vi "Process_data.vi"(4 "Measurement top level?":bool) -> (6 "Vel stat display":string[][](table), 7 "First Plot data Cluster":cluster{"X array":dbl[], "Y array":dbl[]}[](array[cluster]), 8 "Second Plot Data Cluster":cluster{"X array":dbl[], "Y array":dbl[]}[](array[cluster]), 9 "Max Measurement time up":bool)   [LabVIEW 2014]
uses:
  Controls/Inst_type.ctl
  Controls/Instrument_Array.ctl
  Controls/Post_Process.ctl
  Controls/User_Specific_mode.ctl
  Globals/Meas_global.vi
  Globals/LDA_meas_global_1.vi
  Acquisition/PWA/PWAtasksGLOBAL.vi
  Globals/Dynamic_call_global.ph.vi
  Globals/Trav_pos_global.vi
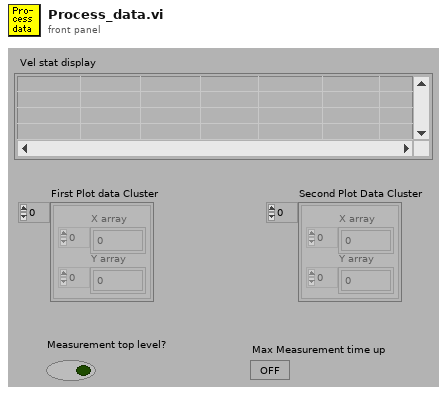
[diagram p1: front panel]
types:
  T1 = typedef "LDA_Setup.ctl" = cluster{"dimensions":enum16{"1D", "2D"}, "Analogue Freq Multiplier":dbl}
  T2 = typedef "PWA_Data.ctl" = enum16{"No PWA Data", "One Ch PWA"}
  T3 = typedef "Inst_type.ctl" = enum16{"Propeller anemometer", "Raw voltage", "Pressure Transducer", "Pitot-static tube", "Preston tube", "Hot wire", "Cross wire 1", "Cross wire 2", "Generic Linear", "Generic Polynomial", "Generic BackPoly", "Fast FID", "Thermocouple", "Cold wire", "Pulsed Wire", "LDA Vel", "LDA Tran time", "LDA Arr time", "Microphone"}
  T4 = typedef "Instrument_Array.ctl" = enum16{"PWA", "LDA", "Analogue"}
  T5 = typedef "Post_Process.ctl" = enum16{"Take New Data", "Post Process Raw Data File"}
  T6 = typedef "User_Specific_mode.ctl" = enum16{"Check VI only", "Run VI"}
  T7 = typedef "Trigger_Mode.ctl" = enum16{"Free Running", "Start on Trigger", "Trigger Every Block", "Trigger Every Sample"}
  T8 = typedef "Analysis_info_cluster.ctl" = cluster{"Colour":u32, "Inst type":T3, "Inst name":string, "Symbol":string, "Code name":string, "Extra Info":string, "Inst Array":T4, "Extra Titles":string[], "Extra Values":string[], "U":dbl, "u^2":dbl, "u^3":dbl, "u^4":dbl, "Skew_u":dbl, "Kurt_u":dbl, "Sd Error in Mean":dbl, "% u'/U":dbl, "X":dbl, "Y":dbl, "Z":dbl, "Timescale integral to 25%":dbl, "Sd Error in Variance":dbl, "Calib File":path, "Calib Constants":dbl[], "Output Position":bool, "Full Stats":bool, "Av Sampling Rate":dbl, "Av No of Samples":dbl, "Total Meas Time (s)":dbl, "ADAM Ch Name":string}
  T9 = typedef "Time_Trace_Cluster.ctl" = cluster{"Weighting":dbl[], "Time (s)":dbl[], "Voltage":dbl[], "Eng Values":dbl[]}
  T10 = typedef "Shift_Cluster.ctl" = cluster{"Stats":dbl[], "Spectra_Auto":dbl[], "Histogram":dbl[], "Hist Max":dbl, "Hist Min":dbl, "No of Samples":i32, "No in plume":i32, "Weigth sum":dbl}
  T11 = typedef "Correlation_cluster1.ctl" = cluster{"U inst":string, "uw":dbl, "u^2w":dbl, "uw^2":dbl, "uw/u'w'":dbl, "W inst":string, "uw^3":dbl, "u^3w":dbl, "u^2w^2":dbl, "Index U":i32, "Index W":i32}
  T12 = typedef "Traverse_cluster.ctl" = cluster{"Start X":sgl, "Start Y":sgl, "Start Z":sgl, "End X":sgl, "End Y":sgl, "End Z":sgl, "No. of pts.":i32, "Spacing":T13, "Filename":path, "Tunnel Speed":dbl, "Averaging time (min)":dbl, "Extra Commands":string, "Carrier_1 Q (l/min)":dbl, "Carrier_2 Q (l/min)":dbl, "Trace Gas Concentration (%)":dbl, "Specific Arguments":string, "Comments":string, "Row No":i32, "Row Type Selector":T14, "Completion time":string, "Row Duration (mins)":dbl, "No. of Valid pts.":i32, "Meas Setup File":string}
  T13 = typedef "Spacing.ctl" = enum16{"Linear", "Log", "Gauss", "Specified", "N/A"}
  T14 = typedef "Multi_run_mode.ctl" = enum16{"Move Traverse Only", "Set Tunnel Speed Only", "Set Source Only", "Set Measurement Conditions", "Single Measurement", "Vertical Profile", "Lateral Profile", "Longitudinal Profile", "Explore Volume", "Multi-Axis Profile", "Auto Calibrate", "Meas Fast FID Bkgnd", "Check Beam Power", "Scanning Valve Measurement", "Run VI Named:", "Set ADAM Ch", "Wait (minutes)", "Send Message", "Synchronize With:", "Fall Back to this Row", "Turn Off Row Repeating", "Blank Row", "Traverse 3D Volume"}
  T15 = typedef "Graph_Type.ctl" = enum16{"Show no graph", "Voltage trace", "Velocity trace", "Vel histogram", "Spectrum", "f.E(f) v Log f", "Auto-Corr"}
  T16 = cluster{"Plot 1":u16, "Plot 2":u16, "Save graph":u16, "Plot Type":T15}
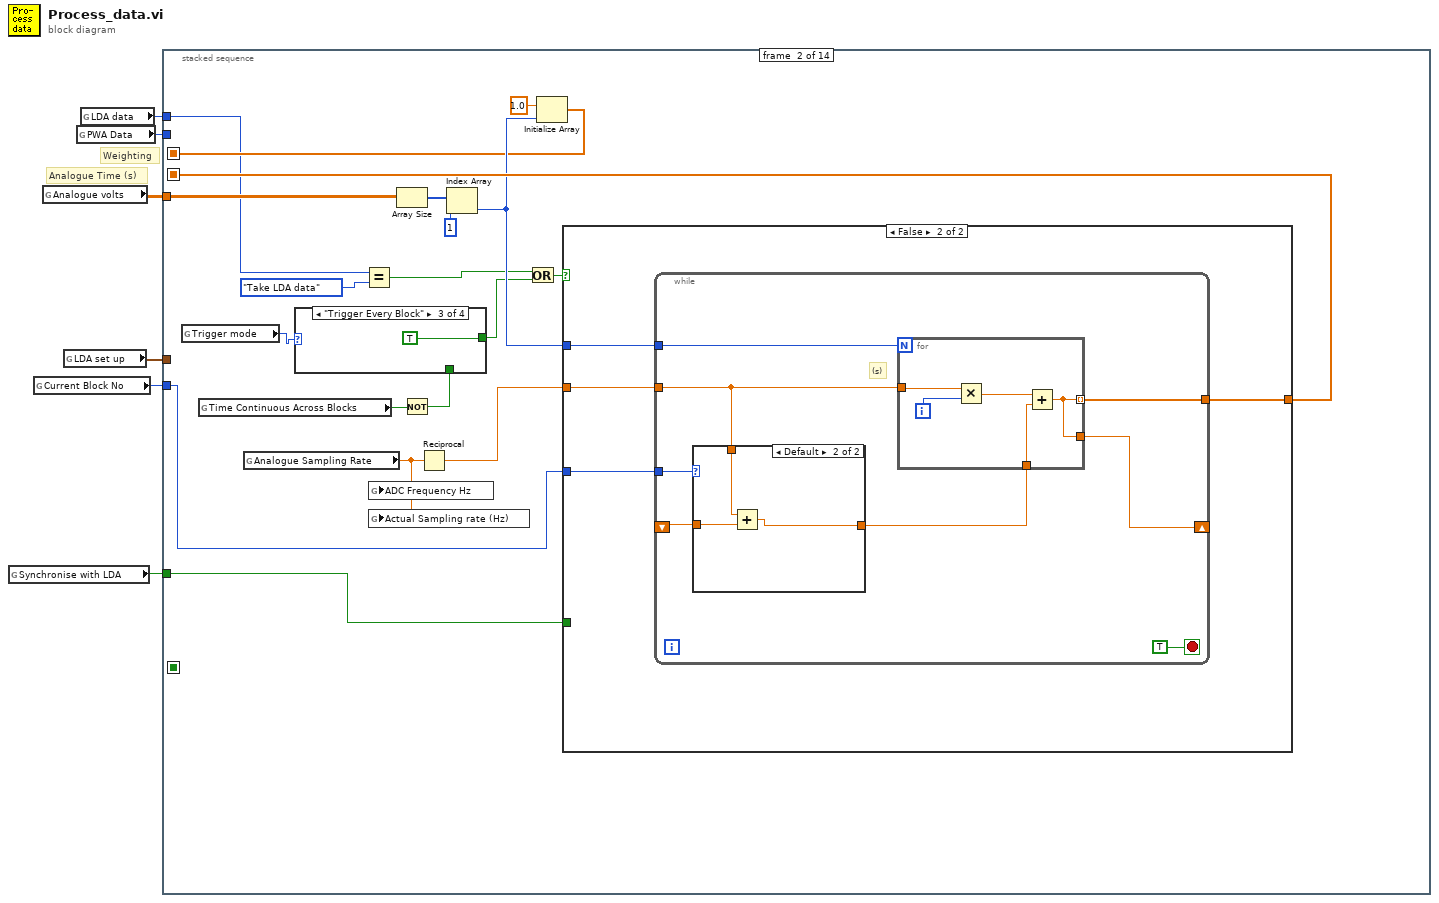
[diagram p0: block diagram]
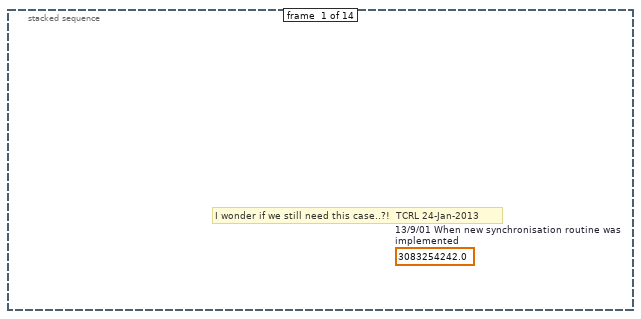
[diagram p2: hidden frame]
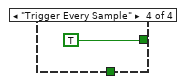
[diagram p5: hidden frame]
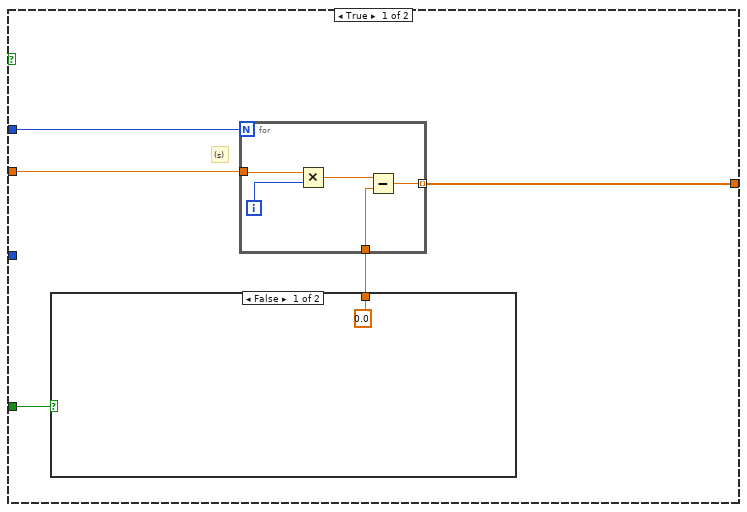
[diagram p6: hidden frame]
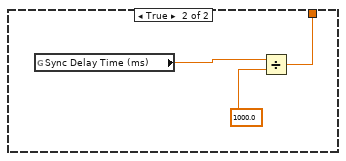
[diagram p7: hidden frame]
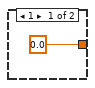
[diagram p8: hidden frame]
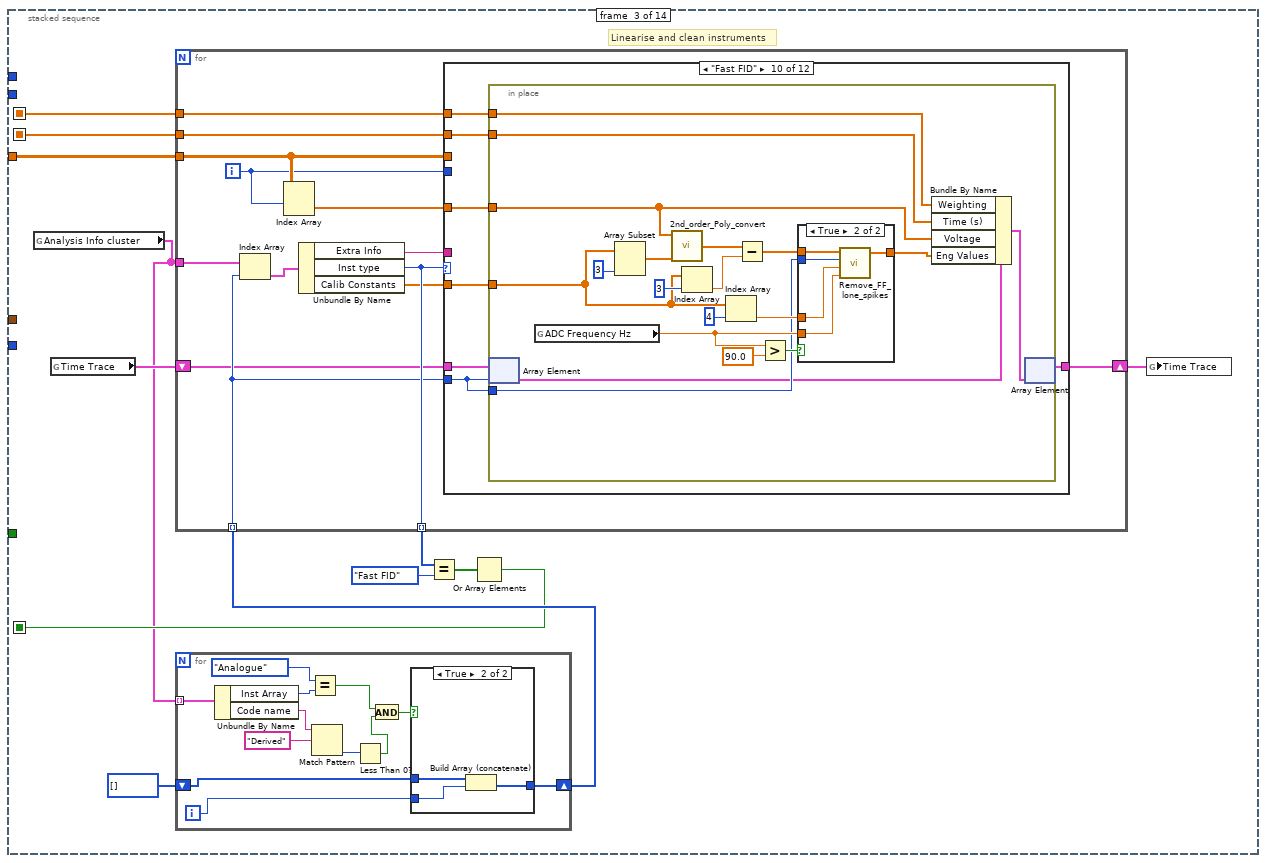
[diagram p9: hidden frame]
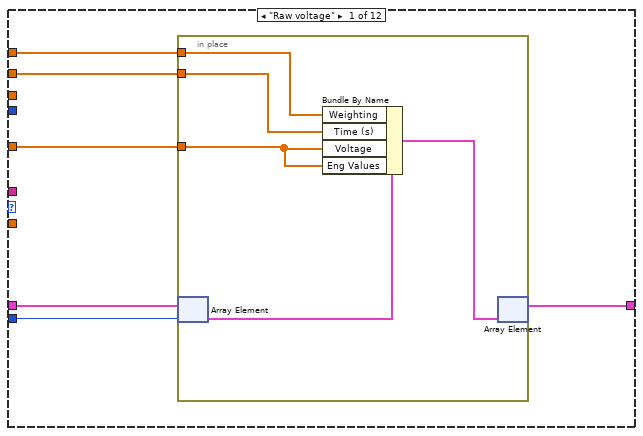
[diagram p11: hidden frame]
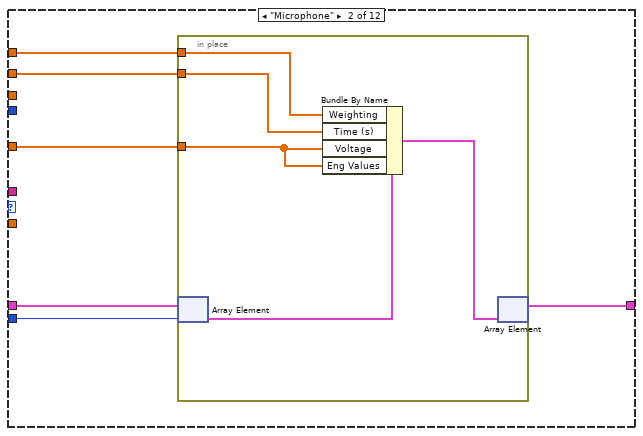
[diagram p12: hidden frame]
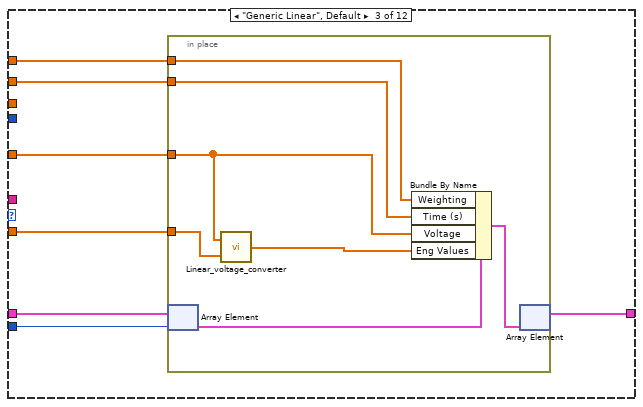
[diagram p13: hidden frame]
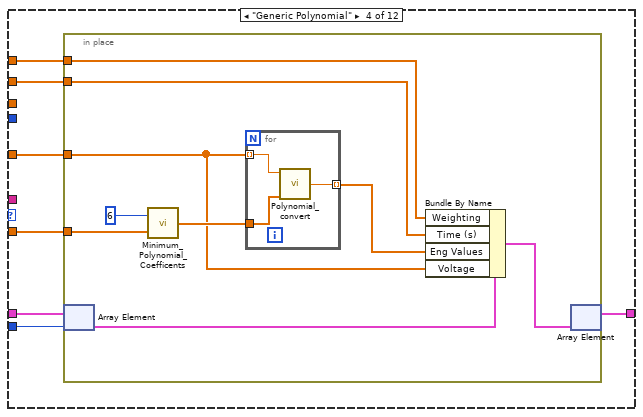
[diagram p14: hidden frame]
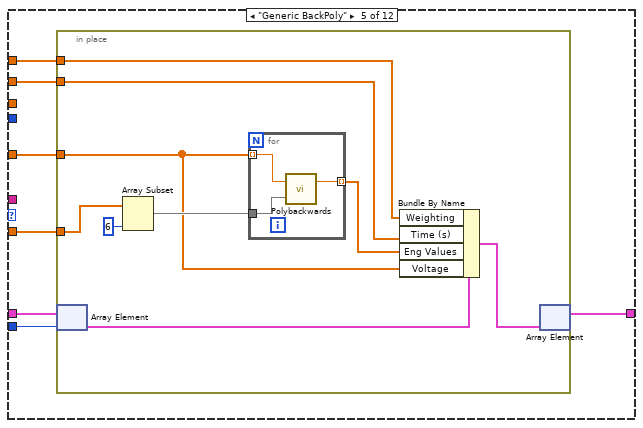
[diagram p15: hidden frame]
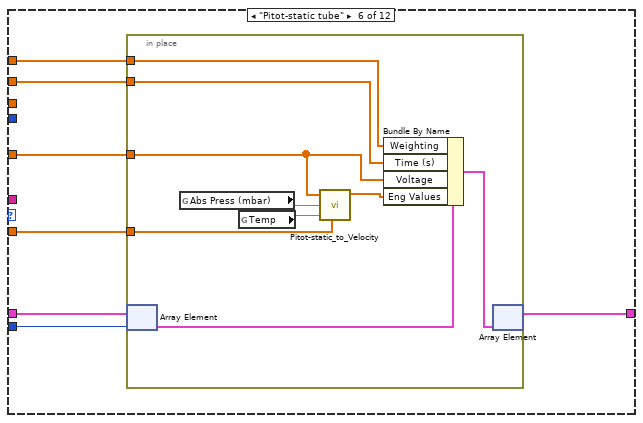
[diagram p16: hidden frame]
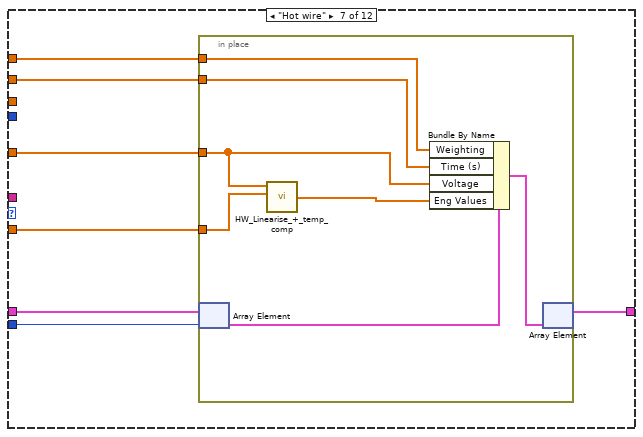
[diagram p17: hidden frame]
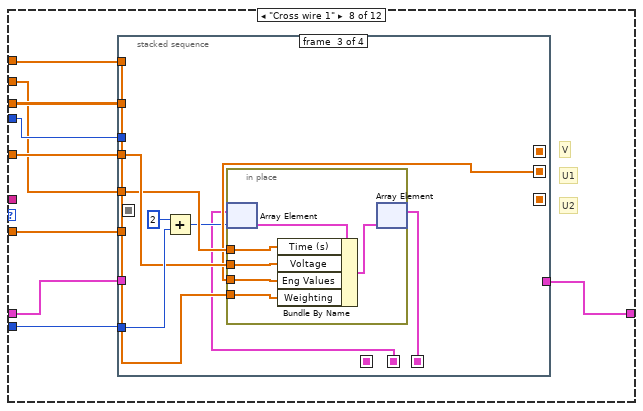
[diagram p18: hidden frame]
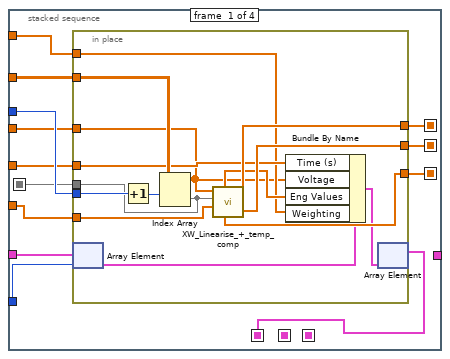
[diagram p19: hidden frame]
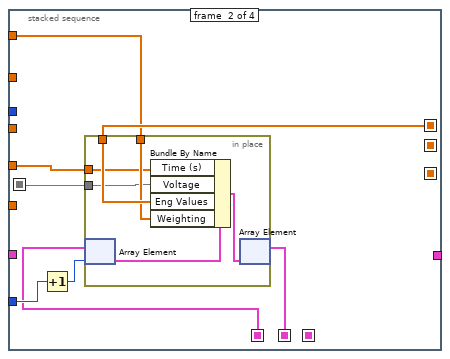
[diagram p20: hidden frame]
diagram:
  # "Weighting"
  # "Analogue Time (s)"
  n1 = global read "Meas_global.vi" "Synchronise with LDA"() -> (w4:bool)
  n2 = global read "Meas_global.vi" "Current Block No"() -> (w5:i32)
  n3 = global read "Meas_global.vi" "Analogue volts"() -> (w2:dbl[][])
  n4 = global read "Meas_global.vi" "LDA set up"() -> (w1:T1)
  n5 = global read "Meas_global.vi" "PWA Data"() -> (w3:T2)
  n6 = global read "Meas_global.vi" "LDA data"() -> (w6:enum16{"No LDA data", "Take LDA data"})
  n7 = stacked-sequence {
    seq-local: [_ w22 _ _ _ _ _ _ _ _ _ _ _ _] -> [_ _ w70 _ _ _ _ _ _ _ _ _ _ _]
    seq-local: [_ w19 _ _ _ _ _ _ _ _ _ _ _ _] -> [_ _ w69 _ _ _ _ _ _ _ _ _ _ _]
    seq-local: [_ _ w66 _ _ _ _ _ _ _ _ _ _ _] -> [_ _ _ _ w431 _ _ _ _ _ _ _ _ _]
    tunnel: w5 -> [_ w15 _ _ _ w435 _ _ _ _ _ _ _ _]
    tunnel: w6 -> [_ w12 _ w385 _ _ _ _ _ _ _ _ _ _]
    tunnel: w2 -> [_ w25 w76 _ _ _ _ _ _ _ _ w644 _ _]
    tunnel: w4 -> [_ w16 _ w384 _ _ _ _ _ _ _ _ _ _]
    tunnel: w3 -> [_ _ _ _ _ w438 _ _ _ _ _ _ _ _]
    tunnel: w1 -> [_ _ _ w382 _ _ _ _ _ _ _ _ _ _]
    frame #0 {
      (unwired) 3083254242.0  # 13/9/01 When new synchronisation routine was implemented
      # "I wonder if we still need this case..?!  TCRL 24-Jan-2013"
    }
    frame #1 {
      n8 = global read "Meas_global.vi" "Trigger mode"() -> (w14:T7)
      n9 = global read "Meas_global.vi" "Time Continuous Across Blocks"() -> (w8:bool)
      n10 = global read "Meas_global.vi" "Analogue Sampling Rate"() -> (w18:dbl)
      n11 = Equal?(x=w12, y=enum16{"No LDA data", "Take LDA data"}."Take LDA data" ("LDA data")) -> (x = y?=w10:bool)
      n12 = global write "LDA_meas_global_1.vi" "ADC Frequency Hz"(w18) -> ()
      n13 = global write "Meas_global.vi" "Actual Sampling rate (Hz)"(w18) -> ()
      n14 = Array Size(array=w25) -> (size(s)=w24:i32[])
      n15 = Not(x=w8) -> (.not. x?=w7:bool)
      n16 = case shown="\"Trigger Every Block\"" w14 {
        tunnel: [w26 w27 TRUE TRUE] -> w9
        tunnel: w7 -> [w26 w27 _ _]
        frame "Free Running" {
        }
        frame "Start on Trigger" {
        }
        frame "Trigger Every Block" {
        }
        frame "Trigger Every Sample" {
        }
      }
      n17 = Reciprocal(x=w18) -> (1/x=w17:dbl)
      n18 = Index Array(array=w24, index=1) -> (element=w21:i32)
      n19 = Or(x=w10, y=w9) -> (x .or. y?=w11:bool)
      n20 = Initialize Array(1.0 ("element"), w21) -> (w19:dbl[])
      n21 = case shown="False" w11 {
        tunnel: [w34 w47] -> w22
        tunnel: w21 -> [w33 w46]
        tunnel: w17 -> [w31 w45]
        tunnel: w16 -> [w30 _]
        tunnel: w15 -> [_ w44]
        frame True {
          # "(s)"
          n22 = case shown="False" w30 {
            tunnel: [0.0 w37] -> w32
            frame False {
            }
            frame True {
              n23 = global read "LDA_meas_global_1.vi" "Sync Delay Time (ms)"() -> (w38:dbl)
              n24 = Divide(x=w38, y=1000.0) -> (x/y=w37:dbl)
            }
          }
          n25 = for {
            N: w33 -> [_]
            tunnel: w31 -> [w42]
            tunnel: [w41] -> w34 mode=indexing
            tunnel: w32 -> [w39]
            i -> [w43]
            n26 = Multiply(x=w42, y=w43) -> (x*y=w40:dbl)
            n27 = Subtract(x=w40, y=w39) -> (x-y=w41:dbl)
          }
        }
        frame False {
          n28 = while {
            tunnel: [w55] -> w47
            tunnel: w46 -> [w54]
            tunnel: w45 -> [w48]
            tunnel: w44 -> [w52]
            shift-right: [w50] -> _
            shift-left: _ -> [w49]
            stop <- TRUE stop-if-true
            # "(s)"
            n29 = case shown="Default" w52 {
              tunnel: [0.0 w57] -> w51
              tunnel: w49 -> [_ w59]
              tunnel: w48 -> [_ w58]
              frame 1 {
              }
              frame Default {
                n30 = Add(x=w58, y=w59) -> (x+y=w57:dbl)
              }
            }
            n31 = for {
              N: w54 -> [_]
              tunnel: w48 -> [w63]
              tunnel: [w60] -> w55 mode=indexing
              tunnel: w51 -> [w61]
              tunnel: [w60] -> w50
              i -> [w64]
              n32 = Multiply(x=w63, y=w64) -> (x*y=w62:dbl)
              n33 = Add(x=w62, y=w61) -> (x+y=w60:dbl)
            }
          }
        }
      }
    }
    frame #2 {
      # "Linearise and clean instruments"
      n34 = global read "Meas_global.vi" "Analysis Info cluster"() -> (w65:T8[])
      n35 = global read "Meas_global.vi" "Time Trace"() -> (w68:T9[])
      n36 = for {
        tunnel: w65 -> [w80] mode=indexing
        shift-right: [w77] -> w71
        shift-left: i32[] [] -> [w78]
        i -> [w79]
        n37 = Unbundle By Name(w80) -> ("Inst Array"=w88:T4, "Code name"=w86:string)
        n38 = Equal?(x=Instrument_Array."Analogue" ("Inst Array"), y=w88) -> (x = y?=w82:bool)
        n39 = Match Pattern(string=w86, regular expression="Derived") -> (offset past match=w84:i32)  [unwired: 4 out]
        n40 = Less Than 0?(x=w84) -> (x < 0?=w83:bool)
        n41 = And(x=w82, y=w83) -> (x .and. y?=w81:bool)
        n42 = case shown="True" w81 {
          tunnel: w79 -> [_ w92]
          tunnel: w78 -> [w89 w91]
          tunnel: [w89 w90] -> w77
          frame False {
          }
          frame True {
            n43 = Build Array (concatenate)(w91, w92) -> (w90:i32[])
          }
        }
      }
      n44 = for {
        tunnel: w76 -> [w104]
        tunnel: [w105] -> w74 mode=indexing
        tunnel: w71 -> [w100] mode=indexing
        shift-right: [w95] -> w67
        shift-left: w68 -> [w99]
        tunnel: w70 -> [w96]
        tunnel: w69 -> [w103]
        tunnel: w65 -> [w102]
        i -> [w94]
        n45 = Index Array(array=w102, index=w100) -> (element=w101:T8)
        n46 = Index Array(array=w104, index (row)=w94) -> (element=w98:dbl[])  [unwired: 1 in]
        n47 = Unbundle By Name(w101) -> ("Extra Info"=w93:string, "Inst type"=w105:T3, "Calib Constants"=w97:dbl[])
        n48 = case shown="\"Fast FID\"" w105 {
          tunnel: w97 -> [_ _ w134 w147 w167 w186 w202 w217 _ w297 w328 w365]
          tunnel: w94 -> [_ _ _ _ _ _ _ w218 _ _ _ _]
          tunnel: w104 -> [_ _ _ _ _ _ _ w215 _ _ _ _]
          tunnel: w96 -> [w106 w117 w128 w146 w163 w180 w196 w212 _ w292 w324 w359]
          tunnel: w98 -> [w107 w118 w133 w148 w166 w185 w201 w216 _ w296 w329 w364]
          tunnel: w100 -> [w110 w121 w132 w144 w164 w182 w197 w214 _ w294 w323 w361]
          tunnel: w99 -> [w111 w122 w130 w143 w165 w183 w199 w213 w290 w295 w327 w362]
          tunnel: [w108 w119 w129 w142 w161 w181 w198 w211 w290 w293 w326 w360] -> w95
          tunnel: w103 -> [w109 w120 w131 w145 w162 w184 w200 w210 _ w291 w325 w363]
          tunnel: w93 -> [_ _ _ _ _ _ _ _ _ _ _ w358]
          frame "Raw voltage" {
            n49 = in-place {
              in-place-border: w109 -> [w112]
              in-place-border: w107 -> [w114]
              in-place-border: w106 -> [w113]
              n50 = in-place-array #1(w111, w110) -> (w115:T9)
              n51 = Bundle By Name(cluster=w115, "Weighting"=w112, "Time (s)"=w113, "Voltage"=w114, "Eng Values"=w114) -> (w116:T9)
              n52 = in-place-array #1(w116) -> (w108:T9[])  [unwired: 1 out]
            }
          }
          frame "Microphone" {
            n53 = in-place {
              in-place-border: w120 -> [w123]
              in-place-border: w118 -> [w125]
              in-place-border: w117 -> [w124]
              n54 = in-place-array #2(w122, w121) -> (w126:T9)
              n55 = Bundle By Name(cluster=w126, "Weighting"=w123, "Time (s)"=w124, "Voltage"=w125, "Eng Values"=w125) -> (w127:T9)
              n56 = in-place-array #2(w127) -> (w119:T9[])  [unwired: 1 out]
            }
          }
          frame "Generic Linear", Default {
            n57 = in-place {
              in-place-border: w134 -> [w141]
              in-place-border: w133 -> [w136]
              in-place-border: w131 -> [w135]
              in-place-border: w128 -> [w137]
              n58 = in-place-array #3(w130, w132) -> (w138:T9)
              n59 = call "Linear_voltage_converter.vi"("Caib const A,B"=w141, "Voltage array"=w136) -> ("Converted array"=w140:dbl[])
              n60 = Bundle By Name(cluster=w138, "Weighting"=w135, "Time (s)"=w137, "Voltage"=w136, "Eng Values"=w140) -> (w139:T9)
              n61 = in-place-array #3(w139) -> (w129:T9[])  [unwired: 1 out]
            }
          }
          frame "Generic Polynomial" {
            n62 = in-place {
              in-place-border: w148 -> [w153]
              in-place-border: w147 -> [w156]
              in-place-border: w146 -> [w150]
              in-place-border: w145 -> [w149]
              n63 = in-place-array #4(w143, w144) -> (w152:T9)
              n64 = call "Minimum_Polynomial_Coefficents.vi"("Calib consts"=w156, "Max Length"=6) -> ("Coefficients"=w155:dbl[])
              n65 = for {
                tunnel: w155 -> [w160]
                tunnel: w153 -> [w159] mode=indexing
                tunnel: [w158] -> w154 mode=indexing
                n66 = call "Polynomial_convert.vi"("Calib constants"=w160, "Voltage"=w159) -> ("Eng Values"=w158:dbl)  [unwired: 4 out]
              }
              n67 = Bundle By Name(cluster=w152, "Weighting"=w149, "Time (s)"=w150, "Eng Values"=w154, "Voltage"=w153) -> (w151:T9)
              n68 = in-place-array #4(w151) -> (w142:T9[])  [unwired: 1 out]
            }
          }
          frame "Generic BackPoly" {
            n69 = in-place {
              in-place-border: w167 -> [w176]
              in-place-border: w166 -> [w171]
              in-place-border: w163 -> [w169]
              in-place-border: w162 -> [w168]
              n70 = in-place-array #5(w165, w164) -> (w173:T9)
              n71 = Array Subset(array=w176, length=6) -> (w175:dbl[])  [unwired: 1 in]
              n72 = for {
                tunnel: w175 -> [w179]
                tunnel: w171 -> [w178] mode=indexing
                tunnel: [w177] -> w172 mode=indexing
                n73 = call "Polybackwards.vi"("Coefficients"=w179, "Y input"=w178) -> ("X output"=w177:dbl)  [unwired: 1 out]
              }
              n74 = Bundle By Name(cluster=w173, "Weighting"=w168, "Time (s)"=w169, "Eng Values"=w172, "Voltage"=w171) -> (w170:T9)
              n75 = in-place-array #5(w170) -> (w161:T9[])  [unwired: 1 out]
            }
          }
          frame "Pitot-static tube" {
            n76 = in-place {
              in-place-border: w186 -> [w195]
              in-place-border: w185 -> [w189]
              in-place-border: w184 -> [w187]
              in-place-border: w180 -> [w190]
              n77 = in-place-array #6(w183, w182) -> (w192:T9)
              n78 = global read "Meas_global.vi" "Abs Press (mbar)"() -> (w194:dbl)
              n79 = global read "Meas_global.vi" "Temp"() -> (w188:dbl)
              n80 = call "Pitot-static_to_Velocity.vi"("Pressure Trans voltage"=w189, "Atmos Press mbar  (1000)"=w194, "Temp  C  (20)"=w188, "Pressure Trans Calib const"=w195) -> ("Velocity (m/s)"=w193:dbl[])  [unwired: 1 in, 3 out]
              n81 = Bundle By Name(cluster=w192, "Weighting"=w187, "Time (s)"=w190, "Voltage"=w189, "Eng Values"=w193) -> (w191:T9)
              n82 = in-place-array #6(w191) -> (w181:T9[])  [unwired: 1 out]
            }
          }
          frame "Hot wire" {
            n83 = in-place {
              in-place-border: w202 -> [w209]
              in-place-border: w201 -> [w204]
              in-place-border: w200 -> [w203]
              in-place-border: w196 -> [w205]
              n84 = in-place-array #7(w199, w197) -> (w207:T9)
              n85 = call "HW_Linearise_+_temp_comp.vi"("Caib const"=w209, "HW voltage"=w204) -> ("Velocity"=w208:dbl[])  [unwired: 3 in, 1 out]
              n86 = Bundle By Name(cluster=w207, "Weighting"=w203, "Time (s)"=w205, "Voltage"=w204, "Eng Values"=w208) -> (w206:T9)
              n87 = in-place-array #7(w206) -> (w198:T9[])  [unwired: 1 out]
            }
          }
          frame "Cross wire 1" {
            # "U2"
            # "U1"
            # "V"
            n88 = stacked-sequence {
              seq-local: [w227 _ _ _] -> [_ w252 _ _]
              seq-local: [w226 _ _ _] -> [_ _ w264 _]
              seq-local: [w225 _ _ _] -> [_ _ _ w280]
              seq-local: [_ w247 _ _] -> [_ _ w261 _]
              seq-local: [_ _ w260 _] -> [_ _ _ w276]
              seq-local: [w224 _ _ _] -> [_ w250 _ w279]
              seq-local: [w221 _ _ _] -> [_ w246 _ _]
              tunnel: w218 -> [w231 _ _ _]
              tunnel: w217 -> [w230 _ _ _]
              tunnel: w216 -> [w229 _ w267 _]
              tunnel: w215 -> [w228 _ _ _]
              tunnel: w214 -> [w222 w253 w268 w283]
              tunnel: w213 -> [w223 _ _ _]
              tunnel: w212 -> [w220 w249 w266 w282]
              tunnel: [_ _ _ w275] -> w211
              tunnel: w210 -> [w219 w251 w263 w278]
              frame #0 {
                n89 = in-place {
                  in-place-border: w231 -> [w245]
                  in-place-border: w230 -> [w243]
                  in-place-border: w229 -> [w232]
                  in-place-border: w228 -> [w242]
                  in-place-border: [w241] -> w227
                  in-place-border: [w240] -> w226
                  in-place-border: [w239] -> w225
                  in-place-border: [w238] -> w224
                  in-place-border: w220 -> [w234]
                  in-place-border: w219 -> [w233]
                  n90 = in-place-array #8(w223, w222) -> (w235:T9)
                  n91 = Increment(x=w245) -> (x+1=w244:i32)
                  n92 = Index Array(array=w242, index (row)=w244) -> (element=w238:dbl[])  [unwired: 1 in]
                  n93 = call "XW_Linearise_+_temp_comp.vi"("Calib const"=w243, "XW2 voltage"=w238, "XW1 voltage"=w232) -> ("U1"=w240:dbl[], "V"=w241:dbl[], "U2"=w239:dbl[], "U"=w237:dbl[])  [unwired: 1 in]
                  n94 = Bundle By Name(cluster=w235, "Time (s)"=w234, "Voltage"=w232, "Eng Values"=w237, "Weighting"=w233) -> (w236:T9)
                  n95 = in-place-array #8(w236) -> (w221:T9[])  [unwired: 1 out]
                }
              }
              frame #1 {
                n96 = Increment(x=w253) -> (x+1=w248:i32)
                n97 = in-place {
                  in-place-border: w252 -> [w259]
                  in-place-border: w251 -> [w258]
                  in-place-border: w250 -> [w257]
                  in-place-border: w249 -> [w256]
                  n98 = in-place-array #9(w246, w248) -> (w255:T9)
                  n99 = Bundle By Name(cluster=w255, "Time (s)"=w256, "Voltage"=w257, "Eng Values"=w259, "Weighting"=w258) -> (w254:T9)
                  n100 = in-place-array #9(w254) -> (w247:T9[])  [unwired: 1 out]
                }
              }
              frame #2 {
                n101 = Add(x=2, y=w268) -> (x+y=w262:i32)
                n102 = in-place {
                  in-place-border: w267 -> [w274]
                  in-place-border: w266 -> [w273]
                  in-place-border: w264 -> [w272]
                  in-place-border: w263 -> [w271]
                  n103 = in-place-array #10(w261, w262) -> (w270:T9)
                  n104 = Bundle By Name(cluster=w270, "Time (s)"=w273, "Voltage"=w274, "Eng Values"=w272, "Weighting"=w271) -> (w269:T9)
                  n105 = in-place-array #10(w269) -> (w260:T9[])  [unwired: 1 out]
                }
              }
              frame #3 {
                n106 = Add(x=3, y=w283) -> (x+y=w277:i32)
                n107 = in-place {
                  in-place-border: w282 -> [w289]
                  in-place-border: w280 -> [w288]
                  in-place-border: w279 -> [w287]
                  in-place-border: w278 -> [w286]
                  n108 = in-place-array #11(w276, w277) -> (w285:T9)
                  n109 = Bundle By Name(cluster=w285, "Time (s)"=w289, "Voltage"=w287, "Eng Values"=w288, "Weighting"=w286) -> (w284:T9)
                  n110 = in-place-array #11(w284) -> (w275:T9[])  [unwired: 1 out]
                }
              }
            }
          }
          frame "Cross wire 2" {
          }
          frame "Fast FID" {
            n111 = in-place {
              in-place-border: w297 -> [w309]
              in-place-border: w296 -> [w300]
              in-place-border: w294 -> [w304]
              in-place-border: w292 -> [w299]
              in-place-border: w291 -> [w298]
              n112 = in-place-array #12(w295, w294) -> (w302:T9)
              n113 = global read "LDA_meas_global_1.vi" "ADC Frequency Hz"() -> (w305:dbl)
              n114 = Array Subset(array=w309, length=3) -> (w308:dbl[])  [unwired: 1 in]
              n115 = call "2nd_order_Poly_convert.vi"("Calib constants"=w308, "Voltage"=w300) -> ("Eng Values"=w307:dbl[])  [unwired: 4 out]
              n116 = Index Array(array=w309, index=3) -> (element=w315:dbl)
              n117 = Index Array(array=w309, index=4) -> (element=w311:dbl)
              n118 = Subtract(x=w307, y=w315) -> (x-y=w314:dbl[])
              n119 = Greater?(x=w305, y=90.0) -> (0:w306:bool)
              n120 = case shown="True" w306 {
                tunnel: w314 -> [w317 w322]
                tunnel: [w317 w321] -> w303
                tunnel: w311 -> [_ w320]
                tunnel: w305 -> [_ w319]
                tunnel: w304 -> [_ w318]
                frame False {
                }
                frame True {
                  n121 = call "Remove_FF_lone_spikes.vi"("ADC Frequency Hz"=w319, "Bkgnd variance"=w320, "AIC index"=w318, "Time Trace"=w322) -> ("Filtered Time Trace"=w321:dbl[])  [unwired: 1 in, 1 out]
                }
              }
              n122 = Bundle By Name(cluster=w302, "Weighting"=w298, "Time (s)"=w299, "Voltage"=w300, "Eng Values"=w303) -> (w301:T9)
              n123 = in-place-array #12(w301) -> (w293:T9[])  [unwired: 1 out]
            }
          }
          frame "Cold wire" {
            n124 = in-place {
              in-place-border: w329 -> [w332]
              in-place-border: w328 -> [w339]
              in-place-border: w325 -> [w330]
              in-place-border: w324 -> [w331]
              n125 = in-place-array #13(w327, w323) -> (w333:T9)
              n126 = call "Minimum_Polynomial_Coefficents.vi"("Calib consts"=w339, "Max Length"=4) -> ("Coefficients"=w338:dbl[])
              n127 = for {
                tunnel: w338 -> [w357]
                tunnel: w332 -> [w356] mode=indexing
                tunnel: [w355] -> w337 mode=indexing
                n128 = call "Polynomial_convert.vi"("Calib constants"=w357, "Voltage"=w356) -> ("Eng Values"=w355:dbl)  [unwired: 4 out]
              }
              n129 = case shown="3" 3 {
                tunnel: w337 -> [w341 w344 w347 w352]
                tunnel: [w341 w343 w345 w351] -> w335
                frame 0, Default {
                }
                frame 3 {
                  n130 = call "Temporary_Cold_Wire_Spike_Replacer.vi"("Data in"=w344, "St Dev threshold"=7.0) -> ("Data out"=w343:dbl[])  [unwired: 1 out]
                }
                frame 1 {
                  n131 = global read "LDA_meas_global_1.vi" "ADC Frequency Hz"() -> (w348:dbl)
                  n132 = Reciprocal(x=w348) -> (1/x=w349:dbl)
                  n133 = call "Ideal_LowPass_Filter_PN.vi"("Cutoff frequency (Hz)"=100.0, "dt (s)"=w349, "1D Data (uniform spacing)"=w347) -> ("Low-pass filtered 1D Data"=w345:dbl[])
                }
                frame 2 {
                  n134 = global read "LDA_meas_global_1.vi" "ADC Frequency Hz"() -> (w353:dbl)
                  n135 = Reciprocal(x=w353) -> (1/x=w354:dbl)
                  n136 = call "Ideal_Notch_Filter_PN.vi"("Frequencies to cut (Hz)"=dbl[] [150.0, 250.0], "dt (s)"=w354, "1D Data (uniform spacing)"=w352) -> ("Low-pass filtered 1D Data"=w351:dbl[])
                }
              }
              n137 = Bundle By Name(cluster=w333, "Weighting"=w330, "Time (s)"=w331, "Voltage"=w332, "Eng Values"=w335) -> (w334:T9)
              n138 = in-place-array #13(w334) -> (w326:T9[])  [unwired: 1 out]
            }
          }
          frame "Preston tube" {
            n139 = in-place {
              in-place-border: w365 -> [w381]
              in-place-border: w364 -> [w368]
              in-place-border: w363 -> [w366]
              in-place-border: w359 -> [w369]
              in-place-border: w358 -> [w367]
              w377 = 0.0  # Static gauge press mm H2O
              n140 = in-place-array #14(w362, w361) -> (w371:T9)
              n141 = global read "Meas_global.vi" "Abs Press (mbar)"() -> (w380:dbl)
              n142 = global read "Meas_global.vi" "Temp"() -> (w374:dbl)
              n143 = Match Pattern(string=w367, regular expression="D = " ("String to match")) -> (after substring=w378:string)  [unwired: 4 out]
              n144 = call "String_2_Number.vi"("Value"=w378) -> ("Numeric"=w373:dbl)
              n145 = Array Size(array=w368) -> (size(s)=w376:i32)
              n146 = call "Preston_shear_stress.vi"("Calib. consts"=w381, "Diam. (mm)"=w373, "Temp (C)"=w374, "Static gauge head mm H2O"=w377, "Atmos. pressure (mbars)"=w380, "Pressure transducer voltages"=w368) -> ("Mean shear stress (Pa)"=w375:dbl)  [unwired: 1 in, 3 out]
              n147 = Initialize Array(w375, w376) -> (w372:dbl[])
              n148 = Bundle By Name(cluster=w371, "Weighting"=w366, "Time (s)"=w369, "Voltage"=w368, "Eng Values"=w372) -> (w370:T9)
              n149 = in-place-array #14(w370) -> (w360:T9[])  [unwired: 1 out]
            }
          }
        }
      }
      n150 = Equal?(x=w74, y=Inst_type."Fast FID" ("Inst type")) -> (x = y?=w73:bool[])
      n151 = Or Array Elements(Boolean array=w73) -> (logical OR=w66:bool)
      n152 = global write "Meas_global.vi" "Time Trace"(w67) -> ()
    }
    frame #3 {
      n153 = Unbundle By Name(w382) -> ("dimensions"=w383:enum16{"1D", "2D"})
      n154 = case shown="\"Take LDA data\"" w385 {
        tunnel: w383 -> [_ w387]
        tunnel: w384 -> [_ w386]
        frame "No LDA data" {
        }
        frame "Take LDA data" {
          # "New Sync"
          n155 = stacked-sequence {
            seq-local: [w391 _ _] -> [_ w394 w396]
            tunnel: w387 -> [_ w395 _]
            tunnel: w386 -> [w392 _ _]
            frame #0 {
              w389 = 3083254242.0  # 13/9/01 When new synchronisation routine was implemented
              n156 = global read "Meas_global.vi" "Time Data was Aquired"() -> (w390:dbl)
              n157 = Greater?(x=w390, y=w389) -> (0:w388:bool)
              n158 = Compound Arithmetic op=AND(w392, w388) -> (w391:bool)
            }
            frame #1 {
              n159 = Not(x=w394) -> (.not. x?=w393:bool)
              n160 = call "LDA_High_Convert_New.vi"("dimensions"=w395, "Create Sync Index"=w393) -> ()  [unwired: 1 in, 4 out]
            }
            frame #2 {
              n161 = case shown="True" w396 {
                frame False {
                }
                frame True {
                  n162 = global read "Meas_global.vi" "Time Trace"() -> (w401:T9[])
                  n163 = global read "Meas_global.vi" "Analysis Info cluster"() -> (w399:T8[])
                  n164 = for {
                    tunnel: w399 -> [w430] mode=indexing
                    tunnel: [w421] -> w402
                    tunnel: w401 -> [w422] mode=indexing
                    stop <- w423 stop-if-true
                    n165 = Unbundle By Name(w422) -> ("Eng Values"=w421:dbl[])
                    n166 = Unbundle By Name(w430) -> ("Inst type"=w428:T3, "Symbol"=w426:string)  [unwired: 1 out]
                    n167 = Equal?(x=Inst_type."Raw voltage" ("Inst type"), y=w428) -> (x = y?=w424:bool)
                    n168 = Equal?(x="Sync", y=w426) -> (x = y?=w425:bool)
                    n169 = And(x=w424, y=w425) -> (x .and. y?=w423:bool)
                  }
                  n170 = global read "Meas_global.vi" "Analogue Sampling Rate"() -> (w405:dbl)
                  n171 = global read "LDA_meas_global_1.vi" "Arrival times"() -> (w403:dbl[])
                  n172 = Reciprocal(x=w405) -> (1/x=w406:dbl)
                  n173 = call "LDA_analogue_start_time_sync_PN.vi"("Correlation peak fit method"=enum32{"Max", "Quadratic", "Gaussian"}."Quadratic", "Pulse high threshold (Volts)"=2.5, "Analogue dt (s)"=w406, "Analogue LDA burst pulse array"=w402, "LDA arrival Times"=w403) -> ("LDA start time rel. to Analogue (s)"=w398:dbl)  [unwired: 3 out]
                  n174 = for {
                    tunnel: w399 -> [w411] mode=indexing
                    tunnel: w398 -> [w412]
                    tunnel: [w410] -> w400 mode=indexing
                    tunnel: w401 -> [w407] mode=indexing
                    n175 = Unbundle By Name(w411) -> ("Inst Array"=w414:T4)
                    n176 = Unbundle By Name(w407) -> ("Time (s)"=w408:dbl[])
                    n177 = Equal?(x=Instrument_Array."LDA" ("Inst Array"), y=w414) -> (x = y?=w409:bool)
                    n178 = case shown="True" w409 {
                      tunnel: w412 -> [_ w420]
                      tunnel: w408 -> [_ w419]
                      tunnel: w407 -> [w415 w418]
                      tunnel: [w415 w416] -> w410
                      frame False {
                      }
                      frame True {
                        n179 = Add(x=w420, y=w419) -> (x+y=w417:dbl[])
                        n180 = Bundle By Name(cluster=w418, "Time (s)"=w417) -> (w416:T9)
                      }
                    }
                  }
                  n181 = global write "Meas_global.vi" "Time Trace"(w400) -> ()
                }
              }
            }
          }
        }
      }
    }
    frame #4 {
      n182 = case shown="True" w431 {
        frame False {
        }
        frame True {
          # "This must not run until the Time trace global has been populated"
          n183 = call "FF_Bkgnd_correction.vi"() -> ()  [unwired: 1 in, 3 out]
        }
      }
    }
    frame #5 {
      n184 = case shown="\"One Ch PWA\"" w438 {
        tunnel: [w440 w452] -> w437
        tunnel: [w440 w451] -> w436
        tunnel: w435 -> [_ w447]
        tunnel: [w439 w445] -> w433
        tunnel: [w439 w444] -> w434
        tunnel: [w439 w442] -> w432
        frame "No PWA Data" {
          w439 = 0 ("y")
          w440 = dbl[][] []
        }
        frame "One Ch PWA" {
          n185 = global read "PWAtasksGLOBAL.vi" "PWA Binary"() -> (w441:i16[][])
          n186 = global read "PWAtasksGLOBAL.vi" "Minimum TOF Index"() -> (w450:i16)
          n187 = global read "PWAtasksGLOBAL.vi" "PWA Lookup Table"() -> (w449:dbl[])
          n188 = Equal?(x=w447, y=1) -> (x = y?=w443:bool)
          n189 = Index Array(array=w441, index (row)=0) -> (element=w455:i16[])  [unwired: 1 in]
          n190 = global read "PWAtasksGLOBAL.vi" "PWA Seconds per clock pulse"() -> (w448:dbl)
          n191 = for {
            tunnel: w455 -> [w474] mode=indexing
            tunnel: [w476] -> w454 mode=indexing
            tunnel: [w475] -> w453 mode=indexing
            tunnel: w450 -> [w473]
            tunnel: w449 -> [w472]
            tunnel: w448 -> [w471]
            shift-right: [w470] -> w445
            shift-left: _ -> [w468]
            shift-right: [w469] -> w444
            shift-left: _ -> [w467]
            tunnel: w443 -> [w464]
            shift-right: [w458] -> w442
            shift-left: _ -> [w460]
            i -> [w466]
            w457 = 0 ("y")
            n192 = Equal To 0?(x=w466) -> (x = 0?=w465:bool)
            n193 = And(x=w464, y=w465) -> (x .and. y?=w461:bool)
            n194 = Select(t=w457, s=w461, f=w460) -> (s? t:f=w459:i32)
            n195 = Select(t=w457, s=w461, f=w468) -> (s? t:f=w463:i32)
            n196 = Select(t=w457, s=w461, f=w467) -> (s? t:f=w462:i32)
            n197 = case shown="0, Default" w474 {
              tunnel: w474 -> [w484 _ _]
              tunnel: [w489 w522 w527] -> w476
              tunnel: [w490 w522 w527] -> w475
              tunnel: w473 -> [w488 _ _]
              tunnel: w472 -> [w486 _ _]
              tunnel: w471 -> [w483 _ _]
              tunnel: w463 -> [w482 w521 w526]
              tunnel: [w481 w520 w525] -> w470
              tunnel: [w479 w519 w524] -> w469
              tunnel: w462 -> [w480 w519 w524]
              tunnel: w459 -> [w478 w518 w523]
              tunnel: [w477 w518 w523] -> w458
              frame 0, Default {
                n198 = Absolute Value(x=w484) -> (abs(x)=w485:i16)
                n199 = Greater?(x=w485, y=w488) -> (0:w487:bool)
                n200 = case shown="True" w487 {
                  tunnel: [w495 w511] -> w490
                  tunnel: [w495 w500] -> w489
                  tunnel: w484 -> [_ w510]
                  tunnel: w486 -> [_ w507]
                  tunnel: w483 -> [_ w505]
                  tunnel: w482 -> [w494 w503]
                  tunnel: [w494 w503] -> w481
                  tunnel: w480 -> [w493 w502]
                  tunnel: [w492 w502] -> w479
                  tunnel: w478 -> [w491 w497]
                  tunnel: [w491 w498] -> w477
                  frame False {
                    w495 = nan
                    n201 = Increment(x=w493) -> (x+1=w492:i32)
                  }
                  frame True {
                    n202 = global read "PWAtasksGLOBAL.vi" "Probe Rotated Thro' 180"() -> (w496:bool)
                    n203 = To Double Precision Float(number=w510) -> (double precision float=w506:dbl)
                    n204 = Add(x=w510, y=i16 4095) -> (x+y=w508:i16)
                    n205 = Multiply(x=w505, y=w506) -> (x*y=w504:dbl)
                    n206 = Index Array(array=w507, index=w508) -> (element=w501:dbl)
                    n207 = Reciprocal(x=w504) -> (1/x=w511:dbl)
                    n208 = case shown="True" w496 {
                      tunnel: w501 -> [w515 w517]
                      tunnel: [w515 w516] -> w500
                      frame False {
                      }
                      frame True {
                        n209 = Negate(x=w517) -> (-x=w516:dbl)
                      }
                    }
                    n210 = Less Than 0?(x=w500) -> (x < 0?=w499:bool)
                    n211 = case shown="True" w499 {
                      tunnel: [w512 w514] -> w498
                      tunnel: w497 -> [w512 w513]
                      frame False {
                      }
                      frame True {
                        n212 = Increment(x=w513) -> (x+1=w514:i32)
                      }
                    }
                  }
                }
              }
              frame 4095 {
                w522 = 0.0 ("Eng Values")
                n213 = Increment(x=w521) -> (x+1=w520:i32)
              }
              frame -4095 {
                w527 = 0.0 ("Eng Values")
                n214 = Increment(x=w526) -> (x+1=w525:i32)
              }
            }
          }
          n215 = Build Array(w453) -> (w452:dbl[][])
          n216 = Build Array(w454) -> (w451:dbl[][])
        }
      }
      n217 = global write "PWAtasksGLOBAL.vi" "PWA 1/TOF"(w437) -> ()
      n218 = global write "PWAtasksGLOBAL.vi" "PWA No of Reverse samples"(w432) -> ()
      n219 = global write "PWAtasksGLOBAL.vi" "PWA No of  TOF Below Min"(w434) -> ()
      n220 = global write "PWAtasksGLOBAL.vi" "PWA No of  TOF Timeouts"(w433) -> ()
      n221 = global write "PWAtasksGLOBAL.vi" "PWA Data"(w436) -> ()
    }
    frame #6 {
      n222 = while {
        shift-right: [w530] -> _
        shift-left: _ -> [w528]
        stop <- FALSE continue-if-true
        n223 = call "Cluster_Analysis.vi"("Shift In"=w528) -> ("Shift Out"=w530:T10[])  [unwired: 2 in]
      }
    }
    frame #7 {
      n224 = global read "Meas_global.vi" "Analysis Info cluster"() -> (w531:T8[])
      n225 = Index Array(array=w531, index=0) -> (element=w540:T8)
      n226 = for {
        tunnel: w531 -> [w568] mode=indexing
        tunnel: [w567] -> w537 mode=indexing
        tunnel: [w555] -> w532 mode=indexing
        n227 = Unbundle By Name(w568) -> ("Total Meas Time (s)"=w555:dbl, "Inst name"=w559:string, "U"=w553:dbl, "u^2"=w562:dbl, "% u'/U"=w565:dbl, "Sd Error in Mean"=w554:dbl, "Full Stats"=w558:bool)
        n228 = call "Number_2_string.vi"("number"=w553) -> ("String"=w560:string)  [unwired: 1 in]
        n229 = call "Number_2_string.vi"("number"=w562) -> ("String"=w561:string)  [unwired: 1 in]
        n230 = Number To Fractional String(number=w565, precision (6)=i16 2) -> (F-format string=w564:string)  [unwired: 2 out]
        n231 = case shown="True" w558 {
          tunnel: [w569 w577] -> w557
          tunnel: [w569 w575] -> w556
          tunnel: w554 -> [_ w572]
          tunnel: w553 -> [_ w571]
          frame False {
            w569 = ""
          }
          frame True {
            n232 = Divide(x=w572, y=w571) -> (x/y=w573:dbl)
            n233 = Multiply(x=w573, y=100.0) -> (x*y=w570:dbl)
            n234 = call "Number_2_string.vi"("number"=w572) -> ("String"=w577:string)  [unwired: 1 in]
            n235 = Number To Fractional String(number=w570, precision (6)=i16 2) -> (F-format string=w575:string)  [unwired: 2 out]
          }
        }
        n236 = Build Array(w559, w560, w561, w564, w557, w556) -> (w563:string[])
        n237 = for {
          tunnel: [w581] -> w567 mode=indexing
          tunnel: w563 -> [w578] mode=indexing
          n238 = Equal?(x="NaN", y=w578) -> (x = y?=w582:bool)
          n239 = Select(t="", s=w582, f=w578) -> (s? t:f=w581:string)
        }
      }
      n240 = Unbundle By Name(w540) -> ("Symbol"=w542:string, "Inst type"=w541:T3)
      n241 = case shown="\"Generic Linear\"" w541 {
        tunnel: ["U" "P" "V" "tau" w587 "C" ("Symbol") "T" ("Symbol") "T" ("Symbol")] -> w539
        tunnel: w542 -> [_ _ _ _ w587 _ _ _]
        frame "Propeller anemometer", Default {
        }
        frame "Pressure Transducer" {
        }
        frame "Raw voltage" {
        }
        frame "Preston tube" {
        }
        frame "Generic Linear" {
        }
        frame "Fast FID" {
        }
        frame "Thermocouple" {
        }
        frame "Cold wire" {
        }
      }
      n242 = To Lower Case(string=w539) -> (all lower case string=w547:string)
      n243 = To Upper Case(1:w539) -> (0:w549:string)
      n244 = Format Into String(format string="%% %s'/%s", w547, w549) -> (resulting string=w548:string)  [unwired: 2 in, 1 out]
      n245 = Concatenate Strings(w547, "^2") -> (w545:string)
      n246 = Build Array("Inst name", w549, w545, w548, "Sd Err in Mean", "% Sd Err") -> (w538:string[])
      n247 = Build Array (concatenate)(w538, w537) -> (w536:string[][])
      n248 = Array Max & Min(array=w532) -> (min value=w533:dbl)  [unwired: 3 out]
      n249 = Divide(x=w533, y=60.0) -> (x/y=w534:dbl)
      n250 = global write "Meas_global.vi" "Vel stat display"(w536) -> ()
      n251 = global write "Meas_global.vi" "Actual Measurement time (min)"(w534) -> ()
    }
    frame #8 {
      n252 = global read "Dynamic_call_global.ph.vi" "Per Block Plug Ins Extra"() -> (w595:string[])
      n253 = global read "Dynamic_call_global.ph.vi" "Per Block Plug Ins"() -> (w596:string[])
      n254 = Build Array (concatenate)(w596, w595) -> (w593:string[])
      n255 = call "Analyse_string_array.vi"("String array"=w593) -> ("Unique strings"=w592:string[])  [unwired: 2 out]
      n256 = Array Size(array=w592) -> (size(s)=w594:i32)
      n257 = Greater Than 0?(x=w594) -> (x > 0?=w591:bool)
      n258 = case shown="True" w591 {
        tunnel: w592 -> [_ w597]
        frame False {
        }
        frame True {
          n259 = call "Call_Block_plug_ins.vi"("Per Block Plug Ins"=w597) -> ()
        }
      }
    }
    frame #9 {
      n260 = while {
        shift-right: [w603] -> _
        shift-left: _ -> [w602]
        stop <- TRUE stop-if-true
        n261 = global read "Meas_global.vi" "Analysis Info cluster"() -> (w604:T8[])
        n262 = global read "Meas_global.vi" "correlate"() -> (w600:i32[][])
        n263 = global read "Meas_global.vi" "Time Trace"() -> (w598:T9[])
        n264 = for {
          tunnel: w600 -> [w619] mode=indexing
          tunnel: w604 -> [w617]
          tunnel: [w615] -> w603 mode=indexing
          tunnel: w602 -> [w614]
          tunnel: [w610] -> w599 mode=indexing
          tunnel: w598 -> [w609]
          i -> [w613]
          n265 = Index Array(array=w614, index (row)=w613) -> (element=w612:dbl[])  [unwired: 1 in]
          n266 = Index Array(array=w619) -> (element #1=w608:i32, element #2=w607:i32)  [unwired: 2 in]
          n267 = Index Array(array=w617, index=w608) -> (element=w618:T8)
          n268 = Index Array(array=w617, index=w607) -> (element=w616:T8)
          n269 = Index Array(array=w609, index=w608) -> (element=w606:T9)
          n270 = Index Array(array=w609, index=w607) -> (element=w605:T9)
          n271 = call "Weighted_Cross_Moments.vi"("AI Cluster 1"=w618, "AI Cluster 2"=w616, "Time Cluster 1"=w606, "Time Cluster 2"=w605, "Shift in"=w612) -> ("output cluster"=w611:T11, "Shift out"=w615:dbl[])  [unwired: 13 in]
          n272 = Bundle By Name(cluster=w611, "Index U"=w608, "Index W"=w607) -> (w610:T11)
        }
        n273 = global write "Meas_global.vi" "Correlation Results"(w599) -> ()
      }
    }
    frame #10 {
      n274 = global read "Meas_global.vi" "Correlation Results"() -> (w624:T11[])
      n275 = global read "Meas_global.vi" "Vel stat display"() -> (w621:string[][])
      n276 = Array Size(array=w624) -> (size(s)=w623:i32)
      n277 = Greater Than 0?(x=w623) -> (x > 0?=w622:bool)
      n278 = case shown="True" w622 {
        tunnel: w624 -> [_ w634]
        tunnel: w621 -> [w625 w627]
        tunnel: [w625 w626] -> w620
        frame False {
        }
        frame True {
          n279 = for {
            tunnel: [w641] -> w629 mode=indexing
            tunnel: w634 -> [w640] mode=indexing
            n280 = Unbundle By Name(w640) -> ("U inst"=w643:string, "W inst"=w642:string, "uw"=w636:dbl, "uw/u'w'"=w638:dbl)
            n281 = call "Number_2_string.vi"("number"=w636) -> ("String"=w635:string)  [unwired: 1 in]
            n282 = Number To Fractional String(number=w638, precision (6)=i16 3) -> (F-format string=w637:string)  [unwired: 2 out]
            n283 = Build Array(w643, w642, w635, w637) -> (w641:string[])
          }
          n284 = Build Array("u inst", "w inst", "uw", "uw/u'w'") -> (w628:string[])
          n285 = Build Array (concatenate)(w627, w628, w629) -> (w626:string[][])
        }
      }
      "Vel stat display" <- w620
      n286 = global write "Meas_global.vi" "Vel stat display"(w620) -> ()
    }
    frame #11 {
      n287 = call "Voltage_overflow_checker.vi"("Voltages"=w644) -> ()  [unwired: 3 out]
    }
    frame #12 {
      # "And declare \"Time's up\" if the error is good enough"
      # "..and the multirun row has valid skip settings in its Extra Commands fiield, and the skip channel has measured long enough to meet its minimum time..."
      # "If we're in a live multirun..."
      n288 = global read "Meas_global.vi" "Post Process"() -> (w649:T5)
      n289 = Equal?(x=w649, y=Post_Process."Take New Data" ("Post Process")) -> (x = y?=w648:bool)
      n290 = global read "Meas_global.vi" "Analysis Info cluster"() -> (w645:T8[])
      n291 = Compound Arithmetic op=AND(w648, invert "Measurement top level?") -> (w646:bool)
      n292 = case shown="True" w646 {
        tunnel: ["" ("Instrument Code Name") w660] -> w654
        tunnel: [0.0 ("Sd Error Theshold value") w659] -> w653
        tunnel: [FALSE w658] -> w651
        frame False {
        }
        frame True {
          n293 = global read "Trav_pos_global.vi" "Current Row"() -> (w661:T12)
          n294 = global read "Meas_global.vi" "Actual Measurement time (min)"() -> (w668:dbl)
          n295 = Unbundle By Name(w661) -> ("Extra Commands"=w662:string)
          n296 = call "Skip_If Sd_Error_Below.vi"("String to Search"=w662, "Simulate/Run"=User_Specific_mode."Run VI", "Measurement setup Applied?"=FALSE) -> ("Check for Skip?"=w666:bool, "Instrument Code Name"=w660:string, "Sd Error Theshold value"=w659:dbl, "Minimum Measurement time (Sec)"=w665:dbl)  [unwired: 2 in, 1 out]
          n297 = Multiply(x=w668, y=60.0) -> (x*y=w670:dbl)
          n298 = Greater Or Equal?(x=w670, y=w665) -> (x >= y?=w667:bool)
          n299 = Compound Arithmetic op=AND(w666, w667) -> (w658:bool)
        }
      }
      n300 = case shown="True" w651 {
        tunnel: w654 -> [_ w675]
        tunnel: w653 -> [_ w674]
        tunnel: [FALSE w673] -> w652
        tunnel: w645 -> [_ w672]
        frame False {
        }
        frame True {
          # "...then check the standard error against the skip threshold"
          n301 = for {
            tunnel: w672 -> [w679] mode=indexing
            tunnel: [w678] -> w676 mode=indexing
            n302 = Unbundle By Name(w679) -> ("Code name"=w681:string)
            n303 = Match Pattern(string=w681, regular expression=":") -> (before substring=w678:string)  [unwired: 4 out]
          }
          n304 = Search 1D Array(1D array=w676, element=w675) -> (index of element=w677:i32)  [unwired: 1 out]
          n305 = case shown="0, Default" w677 {
            tunnel: w677 -> [w687 _]
            tunnel: [w685 FALSE] -> w673
            tunnel: w674 -> [w684 _]
            tunnel: w672 -> [w683 _]
            frame 0, Default {
              n306 = Index Array(array=w683, index=w687) -> (element=w686:T8)
              n307 = Unbundle By Name(w686) -> ("Sd Error in Mean"=w682:dbl)
              n308 = Less?(x=w682, y=w684) -> (x < y?=w685:bool)
            }
            frame -1 {
            }
          }
        }
      }
      "Max Measurement time up" <- w652
    }
    frame #13 {
      n309 = global read "Meas_global.vi" "Second Graph"() -> (w691:T16)
      n310 = global read "Meas_global.vi" "First Graph"() -> (w689:T16)
      n311 = call "Create_Plot.vi"("First Graph"=w689) -> ("Array"=→"First Plot data Cluster":cluster{"X array":dbl[], "Y array":dbl[]}[])
      n312 = call "Create_Plot.vi"("First Graph"=w691) -> ("Array"=→"Second Plot Data Cluster":cluster{"X array":dbl[], "Y array":dbl[]}[])
    }
  }
